vi "findOnTable.vi"(5 "delta":dbl, 7 "table":dbl[][](array[numeric]), 8 "error in (no error)":errorcluster, 9 "column":i32, 10 "key":dbl, 11 "Game in":refnum<class "Game.lvclass">) -> (0 "error out":errorcluster, 2 "search_results":dbl[][](array[numeric]), 3 "Game out":refnum<class "Game.lvclass">)   [LabVIEW 2021, in "Game.lvclass"]
uses:
  Game.lvclass
  25455805-44c3-496a-bc06-ba24b34afc5a.vi
  <vilib>/Array/Sort 2D Array - Pop Stack.vi
  <vilib>/Array/Sort 2D Array - Push Stack.vi
  25455805-44c3-496a-bc06-ba24b34afc5a.vi/269d4b3b-47f5-49e3-8884-44851e4dd9d5.vi
  25455805-44c3-496a-bc06-ba24b34afc5a.vi/6d99389c-673d-4efb-bf33-19b32bcf4cf8.vi
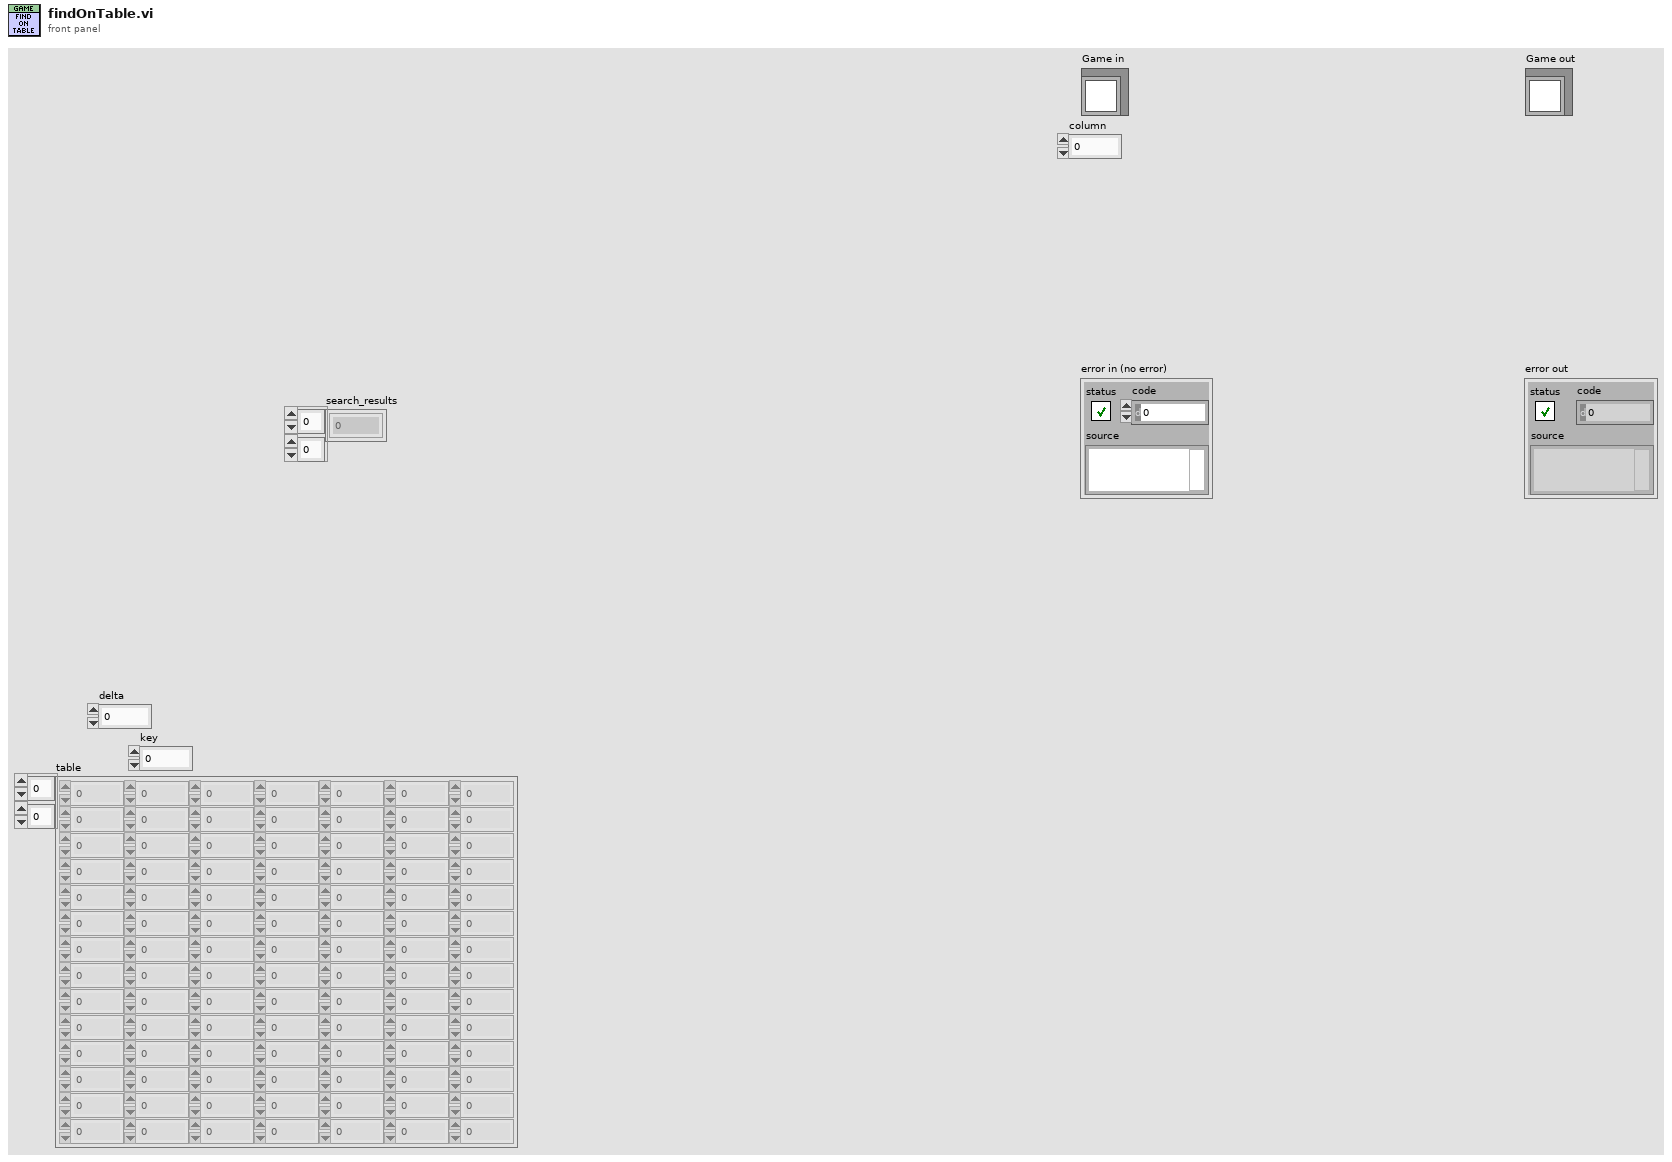
[diagram p1: front panel]
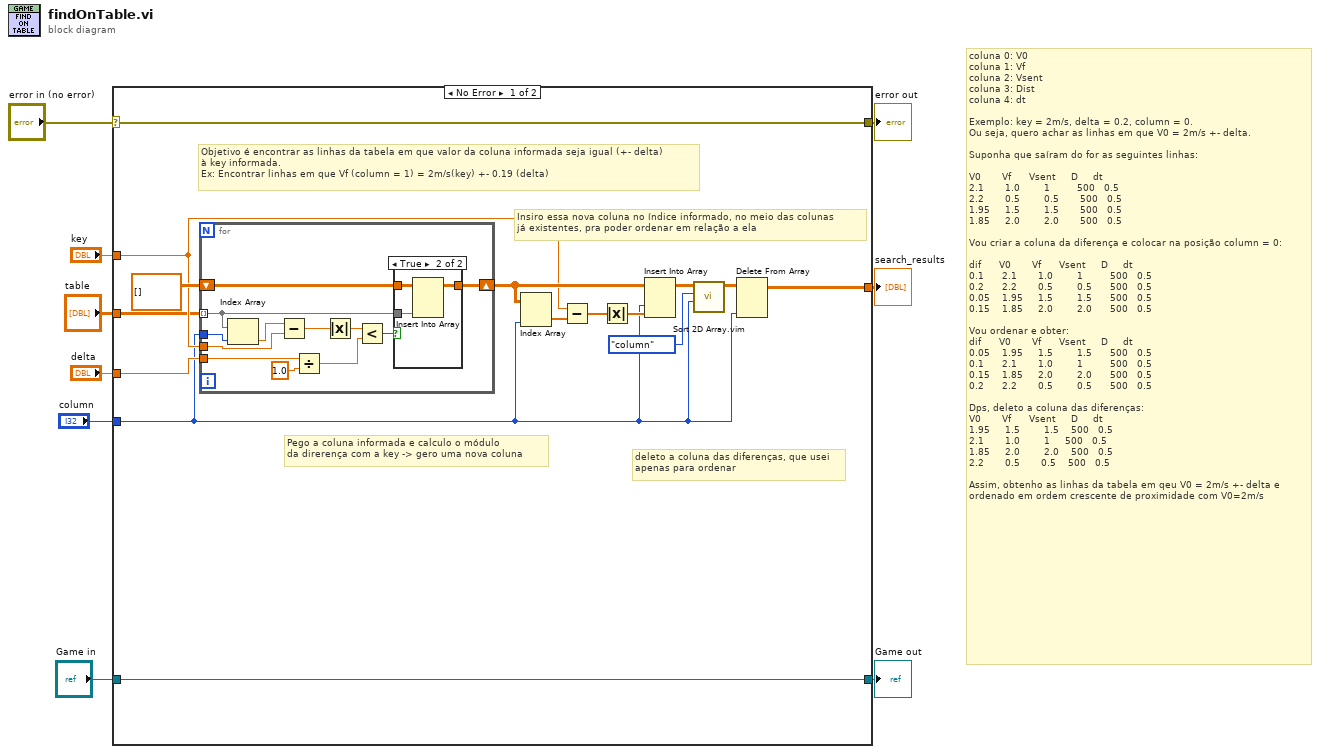
[diagram p0: block diagram]
diagram:
  # "coluna 0: V0\ncoluna 1: Vf\ncoluna 2: Vsent\ncoluna 3: Dist\ncoluna 4: dt\n\nExemplo: key = 2m/s, delta = 0.2, column = 0.\nOu seja, quero achar as linhas em que V0 = 2m/s +- delta.\n\nSuponha que saíram do for as seguintes linhas:\n\nV0       Vf      Vsent     D     dt\n2.1       1.0        1         500   0.5\n2.2       0.5        0.5       500   0.5\n1.95     1.5        1.5       500   0.5\n1.85     2.0        2.0       500   0.5\n\nVou criar a coluna da diferença e colocar na posição column = 0:\n\ndif      V0       Vf      Vsent     D     dt\n0.1      2.1       1.0        1         500   0.5\n0.2      2.2       0.5        0.5      500   0.5\n0.05    1.95     1.5        1.5      500   0.5\n0.15    1.85     2.0        2.0      500   0.5\n\nVou ordenar e obter:\ndif      V0       Vf      Vsent     D     dt\n0.05    1.95     1.5        1.5      500   0.5\n0.1      2.1       1.0        1         500   0.5\n0.15    1.85     2.0        2.0      500   0.5\n0.2      2.2       0.5        0.5      500   0.5\n\nDps, deleto a coluna das diferenças:\nV0       Vf      Vsent     D     dt\n1.95     1.5        1.5    500   0.5\n2.1       1.0        1     500   0.5\n1.85     2.0        2.0    500   0.5\n2.2       0.5       0.5    500   0.5\n\nAssim, obtenho as linhas da tabela em qeu V0 = 2m/s +- delta e\nordenado em ordem crescente de proximidade com V0=2m/s"
  n1 = case shown="No Error" "error in (no error)" {
    selector: "error in (no error)" -> [w23 w42]
    tunnel: [w23 w42] -> w8
    tunnel: [w24 w41] -> w6
    tunnel: "Game in" -> [w24 w41]
    tunnel: "key" -> [w14 _]
    tunnel: "delta" -> [w13 _]
    tunnel: "table" -> [w12 _]
    tunnel: [w11 _] -> w2
    tunnel: "column" -> [w10 _]
    frame No Error {
      # "deleto a coluna das diferenças, que usei\napenas para ordenar"
      # "Insiro essa nova coluna no índice informado, no meio das colunas\njá existentes, pra poder ordenar em relação a ela"
      # "Pego a coluna informada e calculo o módulo\nda direrença com a key -> gero uma nova coluna"
      # "Objetivo é encontrar as linhas da tabela em que valor da coluna informada seja igual (+- delta)\nà key informada.\nEx: Encontrar linhas em que Vf (column = 1) = 2m/s(key) +- 0.19 (delta)"
      n2 = for {
        tunnel: w12 -> [w26] mode=indexing
        tunnel: w14 -> [w36]
        tunnel: w13 -> [w30]
        shift-right: [w31] -> w19
        shift-left: dbl[][] [] ("appended array") -> [w32]
        tunnel: w10 -> [w25]
        n3 = Index Array(array=w26, index=w25) -> (element=w27:dbl)
        n4 = Subtract(x=w27, y=w36) -> (x-y=w35:dbl)
        n5 = Divide(x=w30, y=1.0) -> (x/y=w28:dbl)
        n6 = Absolute Value(x=w35) -> (abs(x)=w34:dbl)
        n7 = Less?(x=w34, y=w28) -> (x < y?=w33:bool)
        n8 = case shown="True" w33 {
          tunnel: w32 -> [w37 w40]
          tunnel: w26 -> [_ w39]
          tunnel: [w37 w38] -> w31
          frame False {
          }
          frame True {
            n9 = Insert Into Array(array=w40, new element=w39) -> (w38:dbl[][])  [unwired: 2 in]
          }
        }
      }
      n10 = Index Array(array=w19, index (col)=w10) -> (element=w16:dbl[])  [unwired: 1 in]
      n11 = Subtract(x=w14, y=w16) -> (x-y=w21:dbl[])
      n12 = Absolute Value(x=w21) -> (abs(x)=w18:dbl[])
      n13 = Insert Into Array(array=w19, index (col)=w10, new element=w18) -> (w17:dbl[][])  [unwired: 1 in]
      n14 = call "Sort 2D Array.vim"("index"=w10, "dimension to index (column)"=enum16{"column", "row"}."column", "2D array"=w17) -> ("sorted 2D array"=w15:dbl[][])  [unwired: 7 in, 1 out]
      n15 = Delete From Array(array=w15, index (col)=w10) -> (array with subset deleted=w11:dbl[][])  [unwired: 2 in, 1 out]
    }
    frame Error {
    }
  }
  "error out" <- w8
  "Game out" <- w6
  "search_results" <- w2
